vi "TabControlToJSON.vi"(8 "error in (no error)":errorcluster, 9 "Owner Bounds":T1, 10 "Folder Path":path, 11 "TabControl in":refnum<vi>) -> (0 "error out":errorcluster, 3 "String out":string)   [LabVIEW 2017]
uses:
  <vilib>/Utility/miscctls.llb/LVRectTypeDef.ctl
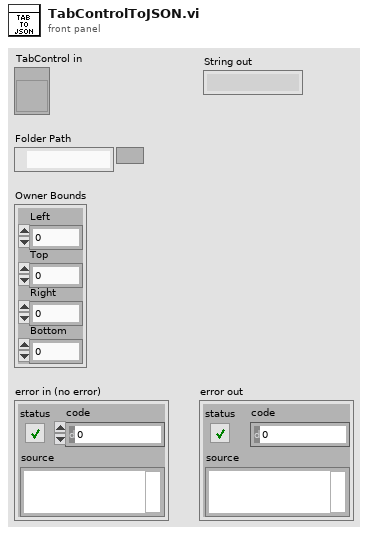
[diagram p1: front panel]
types:
  T1 = typedef "LVRectTypeDef.ctl" = cluster{"Left":i16, "Top":i16, "Right":i16, "Bottom":i16}
  T2 = typedef "LVBoundsTypeDef.ctl" = cluster{"Width":u32, "Height":u32}
  T3 = typedef "imagedata.ctl" = cluster{"image type":i32, "image depth":i32, "image":u8[], "mask":u8[], "colors":u32[], "Rectangle":cluster{"left":i16, "top":i16, "right":i16, "bottom":i16}}
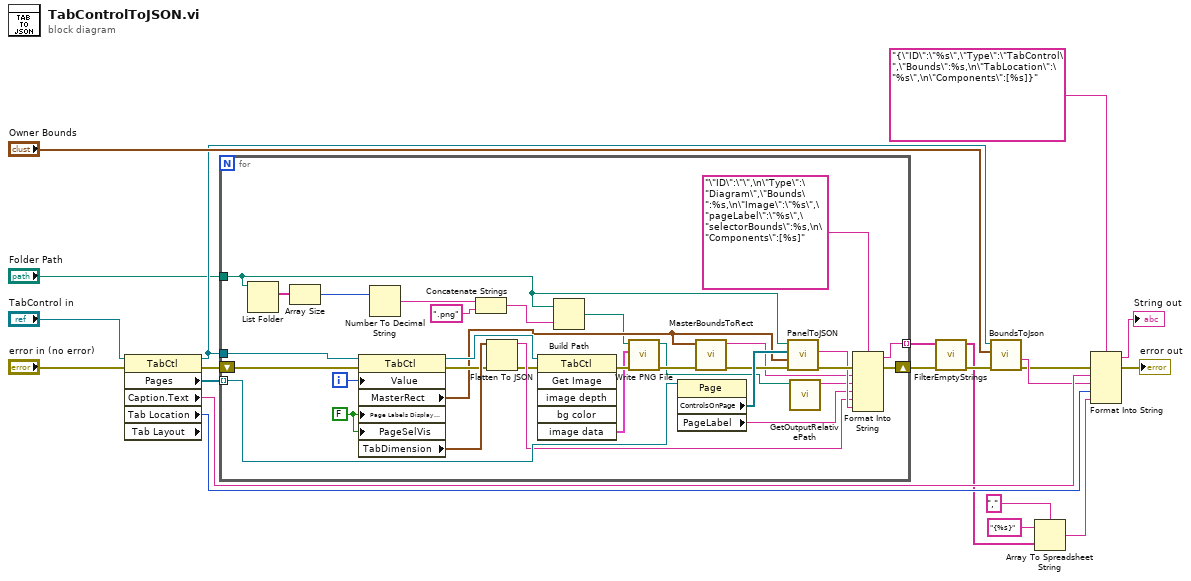
[diagram p0: block diagram]
diagram:
  n1 = property class="TabCtl" props=["Pages", "Caption", "Text", "Tab Location", "Tab Layout"](reference="TabControl in", error in="error in (no error)") -> (reference out=w12:refnum<vi>, error out=w16:errorcluster, "Pages"=w3:refnum<vi>[], "Caption.Text"=w19:string, "Tab Location"=w20:enum32{"Top", "Bottom", "Left", "Right"})  [unwired: 1 out]
  n2 = for {
    tunnel: w12 -> [w43]
    tunnel: w3 -> [w51] mode=indexing
    tunnel: "Folder Path" -> [w27]
    tunnel: [w49] -> w9 mode=indexing
    shift-right: [w36] -> w17
    shift-left: w16 -> [w37]
    i -> [w42]
    w35 = FALSE
    n3 = List Folder(path=w27) -> (filenames=w30:string[])  [unwired: 3 in, 3 out]
    n4 = Array Size(array=w30) -> (size(s)=w28:i32)
    n5 = property class="TabCtl"(reference=w43, error in=w37, "Value"=w42, "Page Labels Display Visible?"=w35, "PageSelVis"=w35) -> (reference out=w44:refnum<vi>, error out=w39:errorcluster, "MasterRect"=w31:T1, "TabDimension"=w41:T2)
    n6 = Number To Decimal String(number=w28) -> (decimal integer string=w29:string)  [unwired: 1 in]
    n7 = Concatenate Strings(w29, ".png" ("string")) -> (w26:string)
    n8 = Flatten To JSON(anything=w41, error in (no error)=w39) -> (JSON string=w40:string, 11:w38:errorcluster)  [unwired: 1 in]
    n9 = invoke class="TabCtl" method="Get Image"(reference=w44, error in=w38) -> (error out=w53:errorcluster, "image data"=w48:T3)  [unwired: 4 in, 4 out]
    n10 = Build Path(base path=w27, name or relative path=w26) -> (appended path=w25:path)
    n11 = call <vilib>:"Write PNG File.vi"("error in (no error)"=w53, "image data"=w48, "path to PNG file"=w25) -> ("error out"=w34:errorcluster, "path"=w23:path)  [unwired: 7 in]
    n12 = property class="Page"(reference=w51) -> ("ControlsOnPage"=w50:refnum<vi>[], "PageLabel"=w24:string)  [unwired: 1 in, 2 out]
    n13 = call "MasterBoundsToRect.vi"("error in"=w34, "Owner Bounds"=w31) -> ("error out"=w33:errorcluster, "JSON"=w32:string)  [unwired: 8 in]
    n14 = call "PanelToJSON.vi"("error in (no error)"=w33, "Owner Bounds"=w31, "Controls[]"=w50, "Folder Path"=w27) -> ("error out"=w47:errorcluster, "spreadsheet string"=w45:string)  [unwired: 6 in]
    n15 = call "GetOutputRelativePath.vi"("Path"=w23) -> ("Output relative path"=w22:string)  [unwired: 9 in, 1 out]
    n16 = Format Into String(format string="\"ID\":\"\",\n\"Type\":\"Diagram\",\"Bounds\":%s,\n\"Image\":\"%s\",\"pageLabel\":\"%s\",\"selectorBounds\":%s,\n\"Components\":[%s]", error in=w47, w32, w22, w24, w40, w45) -> (resulting string=w49:string, error out=w36:errorcluster)  [unwired: 1 in]
  }
  n17 = call "FilterEmptyStrings.vi"("error in"=w17, "Array in"=w9) -> ("error out"=w13:errorcluster, "Array out"=w10:string[])  [unwired: 8 in]
  n18 = call "BoundsToJson.vi"("error in (no error)"=w13, "Owner Bounds"="Owner Bounds", "GObj in"=w12) -> ("error out"=w14:errorcluster, "JSON"=w18:string)  [unwired: 5 in, 2 out]
  n19 = Array To Spreadsheet String(delimiter (Tab)=",", array=w10, 3:"{%s}" ("format string")) -> (spreadsheet string=w11:string)
  n20 = Format Into String(format string="{\"ID\":\"%s\",\"Type\":\"TabControl\",\"Bounds\":%s,\n\"TabLocation\":\"%s\",\n\"Components\":[%s]}", error in=w14, w19, w18, w20, w11) -> (resulting string=→"String out":string, error out=→"error out":errorcluster)  [unwired: 1 in]
